vi "Check Status.vi"(8 "error in (no error)":errorcluster, 11 "Dummy in":refnum<class "Dummy.lvclass">) -> (0 "error out":errorcluster, 1 "Status":string, 2 "Ready?":bool, 3 "Dummy out":refnum<class "Dummy.lvclass">)   [LabVIEW 2017, in "Dummy.lvclass"]
doc: "(Dynamic) Check if the instrument is powered on and update its member fields with the instrument's current status. Optionally return a text status message."
uses:
  Dummy.lvclass
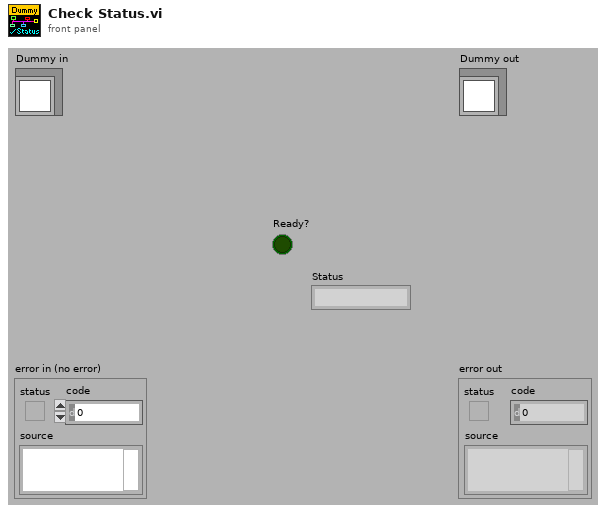
[diagram p1: front panel]
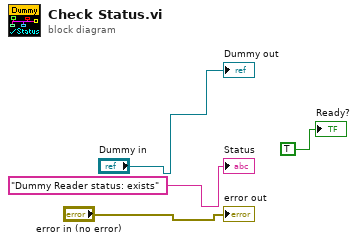
[diagram p0: block diagram]
diagram:
  "error out" <- "error in (no error)"
  "Dummy out" <- "Dummy in"
  "Status" <- "Dummy Reader status: exists" ("Status")
  "Ready?" <- TRUE ("Ready?")
